vi "Starter Kit 2.0 FPGA Globals.vi"() -> ()   [LabVIEW 2013]
panel:
  in  "velocity interval (ticks)":u32=640000
  out "DCmotor_1_ppi vel":i32
  out "DCmotor_0_ppi vel":i32
  # "640000 ticks = 16 ms"
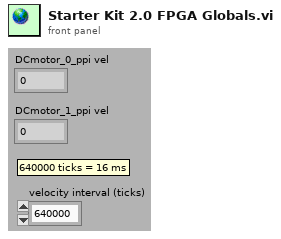
[diagram p1: front panel]
diagram:
